vi "Write Light Stack State.vi"(8 "error in":errorcluster, 9 "State":T1, 10 "Light Select":T2, 11 "PLC in":refnum<class "PLC.lvclass">) -> (0 "error out":errorcluster, 3 "PLC out":refnum<class "PLC.lvclass">)   [LabVIEW 2018, in "PLC.lvlib" / "PLC.lvclass"]
uses:
  PLC.lvclass
  PPLs/PLC/Light Stack/Light Stack.lvlibp/Custom Controls/Light Select.ctl
  PPLs/PLC/Light Stack/Light Stack.lvlibp/Custom Controls/Light Mode.ctl
  Custom Controls/Selector.ctl
  PLC.lvclass/PLC.ctl
  PPLs/PLC/Light Stack/Light Stack.lvlibp/Light Stack.lvclass
  PPLs/PLC/Light Stack/Light Stack.lvlibp
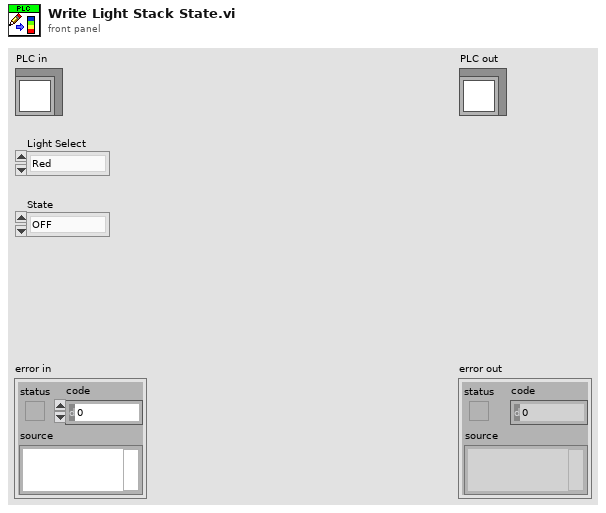
[diagram p1: front panel]
types:
  T1 = typedef "Light Stack.lvlibp/Light Mode.ctl" = enum16{"OFF", "ON", "BLINK"}
  T2 = typedef "Light Stack.lvlibp/Light Select.ctl" = enum16{"Red", "Amber", "Green", "Blue"}
  T3 = typedef "PLC.lvlib/PLC.lvclass/Selector.ctl" = enum16{"Digital", "Analog"}
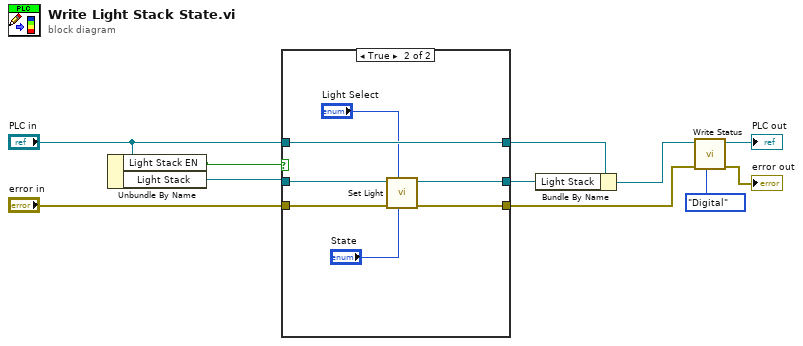
[diagram p0: block diagram]
diagram:
  n1 = Unbundle By Name("PLC in") -> ("Light Stack EN"=w6:bool, "Light Stack"=w5:refnum<class "Light Stack.lvclass">)
  n2 = case shown="True" w6 {
    tunnel: [w14 w21] -> w4
    tunnel: "PLC in" -> [w14 w21]
    tunnel: w5 -> [w13 w20]
    tunnel: "error in" -> [w12 w19]
    tunnel: [w13 w17] -> w2
    tunnel: [w12 w18] -> w1
    frame False {
    }
    frame True {
      n3 = call "Set Light.vi"("State"="State", "Light Select"="Light Select", "error in"=w19, "Light Stack in"=w20) -> ("error out"=w18:errorcluster, "Light Stack out"=w17:refnum<class "Light Stack.lvclass">)  [unwired: 6 in]
    }
  }
  n4 = Bundle By Name(cluster=w4, "Light Stack"=w2) -> (w3:refnum<class "PLC.lvclass">)
  n5 = call-dynamic "Write Status.vi"("Selector"=Selector."Digital", "error in"=w1, "PLC in"=w3) -> ("error out"=→"error out":errorcluster, "PLC out"=→"PLC out":refnum<class "PLC.lvclass">)  [unwired: 7 in]
